vi "Add_Props_Colormap.vi"(10 "Colormap":T2={"Map"=enum."Automatic", "Value Min"=nan, "Value Max"=nan, "Scaling"=enum."Default", "Reverse"=FALSE}, 11 "Keyword Array":T1[](array[typedef])) -> (3 "Keyword Array Out":T1[](array[typedef]))   [LabVIEW 2013, in "Advanced Plotting Toolkit.lvlib"]
uses:
  Advanced Plotting Toolkit.lvlib
  properties/Colormap.ctl
  properties/Colormap_Map.ctl
  properties/Colormap_Scaling.ctl
  KeyValue.ctl
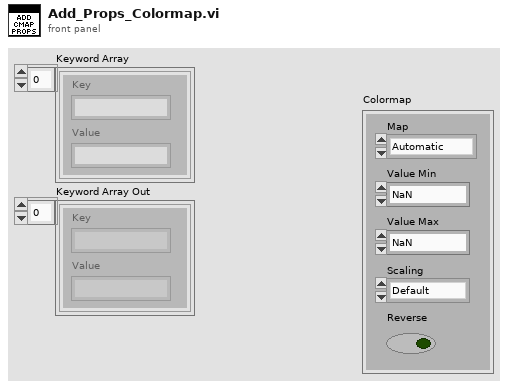
[diagram p1: front panel]
types:
  T1 = typedef "Advanced Plotting Toolkit.lvlib/KeyValue.ctl" = cluster{"Key":string, "Value":string}
  T2 = typedef "Advanced Plotting Toolkit.lvlib/Colormap.ctl" = cluster{"Map":T3, "Value Min":dbl, "Value Max":dbl, "Scaling":T4, "Reverse":bool}
  T3 = typedef "Advanced Plotting Toolkit.lvlib/Colormap_Map.ctl" = enum16{"Automatic", "Rainbow", "Hot and Cold", "White-Black", "White-Blue", "White-Green", "White-Red", "Fire", "Water", "Earth", "Air", "Pastel", "Banded", "Stepped"}
  T4 = typedef "Advanced Plotting Toolkit.lvlib/Colormap_Scaling.ctl" = enum16{"Default"}
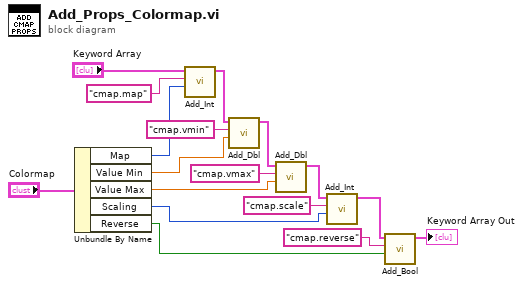
[diagram p0: block diagram]
diagram:
  n1 = Unbundle By Name("Colormap") -> ("Map"=w14:T3, "Value Min"=w11:dbl, "Value Max"=w10:dbl, "Scaling"=w5:T4, "Reverse"=w1:bool)
  n2 = call "Add_Int.vi"("Value"=w14, "Key"="cmap.map", "Keyword Array"="Keyword Array") -> ("Keyword Array Out"=w12:T1[])  [unwired: 8 in]
  n3 = call "Add_Dbl.vi"("Value"=w11, "Key"="cmap.vmin", "Keyword Array"=w12) -> ("Keyword Array Out"=w9:T1[])  [unwired: 8 in]
  n4 = call "Add_Dbl.vi"("Value"=w10, "Key"="cmap.vmax", "Keyword Array"=w9) -> ("Keyword Array Out"=w7:T1[])  [unwired: 8 in]
  n5 = call "Add_Int.vi"("Value"=w5, "Key"="cmap.scale", "Keyword Array"=w7) -> ("Keyword Array Out"=w4:T1[])  [unwired: 8 in]
  n6 = call "Add_Bool.vi"("Value"=w1, "Key"="cmap.reverse", "Keyword Array"=w4) -> ("Keyword Array Out"=→"Keyword Array Out":T1[])  [unwired: 8 in]
